vi "THzTime_SPEED_control_for Varying Gap_170120.vi"(1 "ESP300 Axis":i8=1, 2 "ESP300 Address":string="1", 4 "Lockin Address":string="12") -> ()   [LabVIEW 2010]
panel:
  in  "?":bool
  out "Current Round":i32=100
  out "Current Gap (um)":u32=50
  in  "Initial Gap (um)":u32=50
  out "error out":errorcluster
  in  "Number of Gap":u32=5
  in  "Number of Avg":u32=50
  in  "Gap Increase (um)":u32=25
  in  "Step Increase (um)":u32=5
  in  "error in (no error)":errorcluster
  in  "MCS System Locator":string="usb:id:1441320285"
  out "Y position":dbl=-0.3427166666666667 format="%#.3p"
  out "X position":dbl=-0.44846666666666674 format="%#.3p"
  out "Power meter":dbl=48.63333333333333 format="%#.3p"
  in  "Save File Name":string="vg_"
  in  "Launch server?":bool
  in  "Authorize?":bool=TRUE
  in  "CONEX-PSD9 Instrument Key 2":string="CONEX-PSD (A6ULD73M)"
  in  "Interdelay (ms)":dbl=20.0
  in  "pre delay(ms)":dbl=300.0
  out "Lock-in Y-Channel":dbl=7.27601e-12 format="%#.3p"
  out "Lock-in X-Channel":dbl=7.27601e-12 format="%#.3p"
  out "THz Time-domain Signal Wave":cluster{"x-axis":sgl[], "y-axis":dbl[]}(graph)
  in  "Autosave Directory for Long-term Average Scan":path=path "D:/taianh/Measurement Data/170121 Variable Gap"
  out "Phase":cluster{"f0":dbl, "df":dbl, "magnitude":dbl[]}(graph)
  in  "OK Button":bool
  out "Data Type":string="outp ? 1"
  in  "Enum":enum16{"X", "Y", "Abs"}(ring)
  in  "Draw":bool
  in  "Exit Program":bool
  out "Amplitude":cluster{"f0":dbl, "df":dbl, "magnitude":dbl[]}(graph)
  in  "Short term \nAverage#":i8=1
  in  "Step":sgl=0.005 min=0 max=10000 format="%.3f"
  in  "End Position":sgl=-18.5 min=-75 max=75 format="%#.3f"
  in  "Start Position":sgl=-16.2 min=-75 max=75 format="%#.3f"
  # "Data"
  # "Auto-offset"
  # "Start Position (mm)"
  # "End Position (mm)"
  # "Step (mm)"
  # "Point Avg"
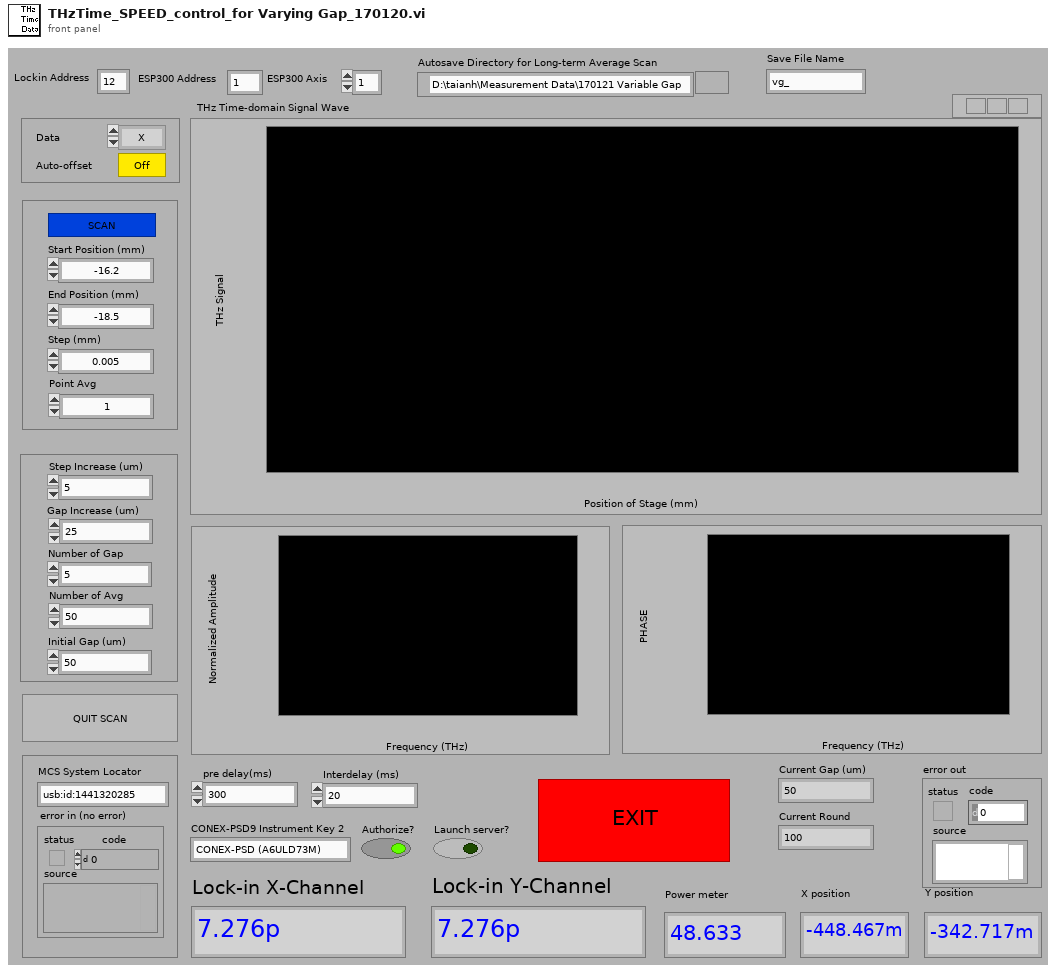
[diagram p1: front panel]
types:
  T1 = cluster{"ConexPSD Reference":refnum<k24>, "error out":errorcluster, "Component ID":i32}
  T2 = cluster{"System Index Out":u32, "error out":errorcluster}
  T3 = cluster{"Step Number":i32, "Step":sgl, "Start Position":sgl, "Time-out":i32, "Lockin Address":string, "Short term \nAverage#":i8, i32, "ESP300 Axis":i8, "Value":string, "pre delay(ms)":dbl, "Interdelay (ms)":dbl, "Autosave Directory for Long-term Average Scan":path, cluster{"ConexPSD Reference":refnum<k24>, "error out":errorcluster, "Component ID":i32}}
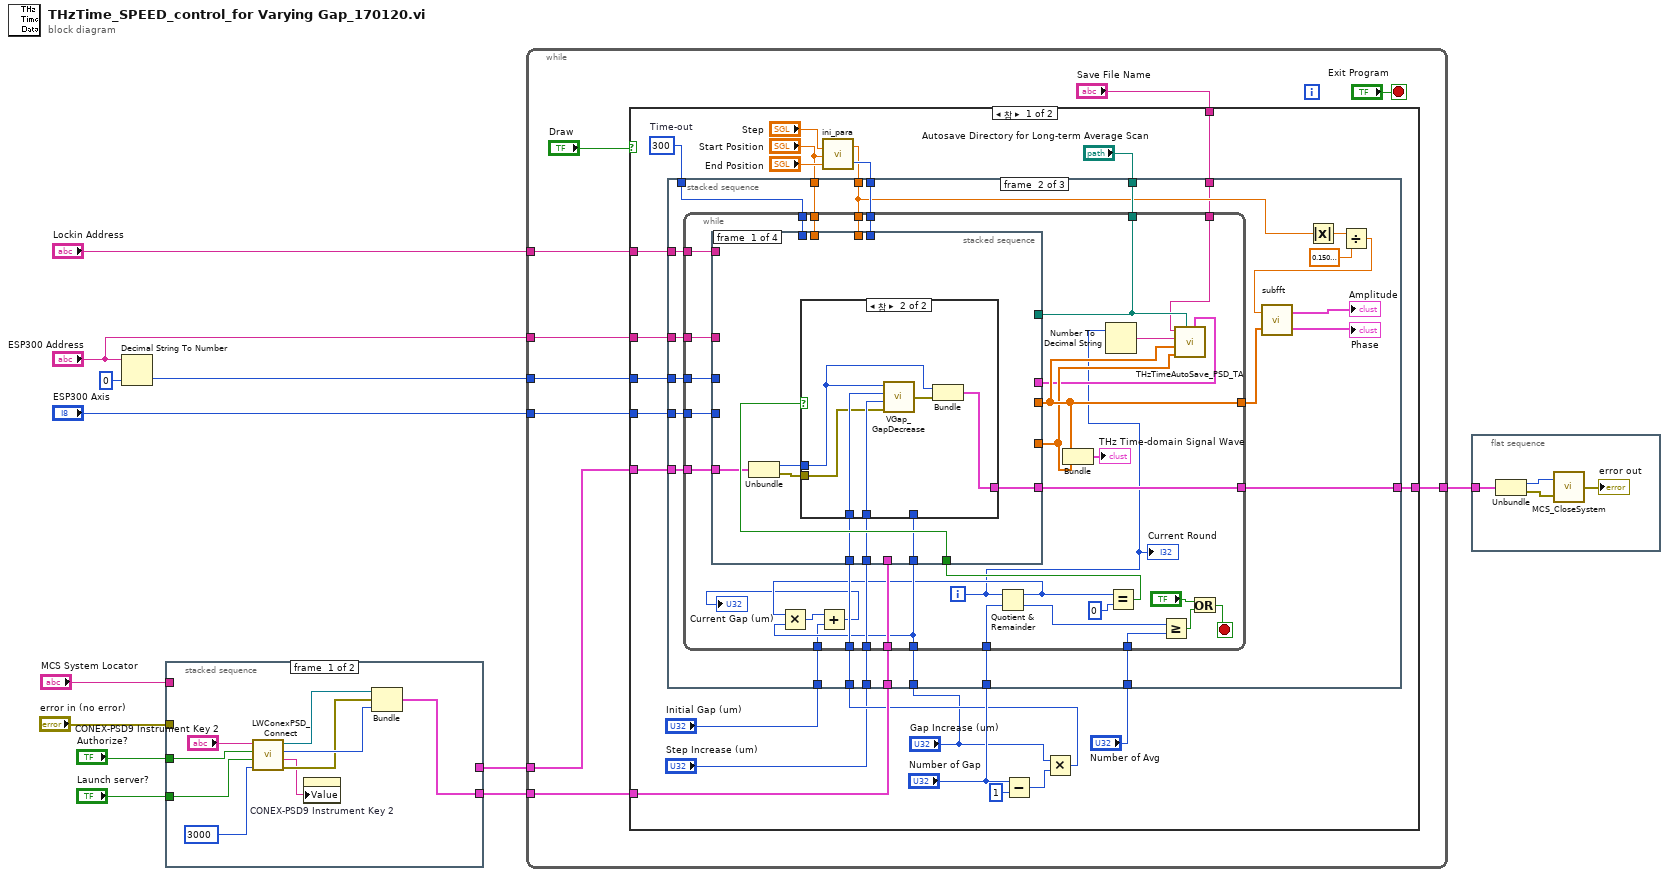
[diagram p0: block diagram]
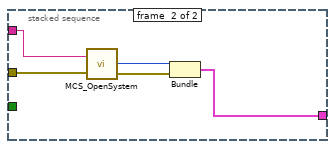
[diagram p2: hidden frame]
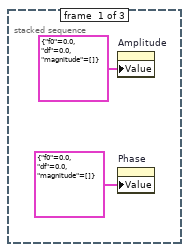
[diagram p3: hidden frame]
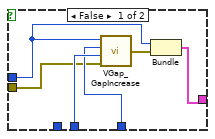
[diagram p4: hidden frame]
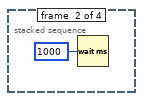
[diagram p5: hidden frame]
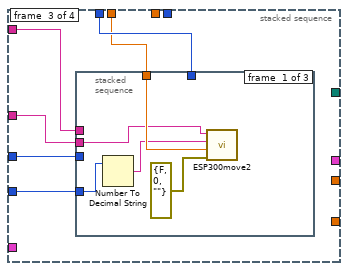
[diagram p6: hidden frame]
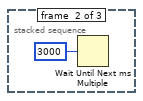
[diagram p7: hidden frame]
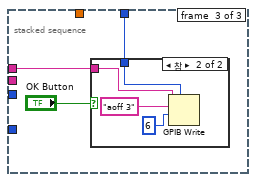
[diagram p8: hidden frame]
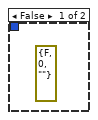
[diagram p9: hidden frame]
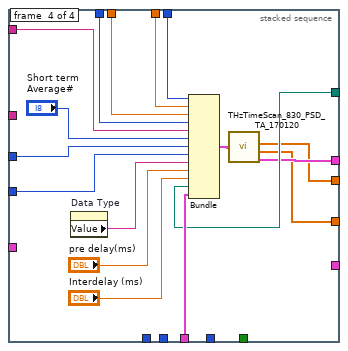
[diagram p10: hidden frame]
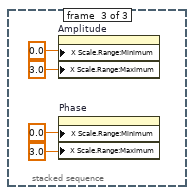
[diagram p11: hidden frame]
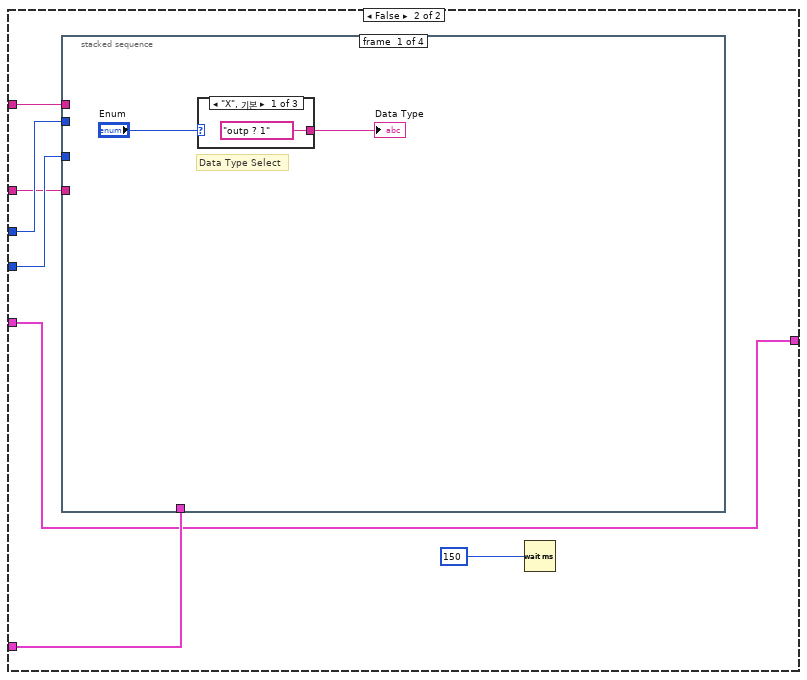
[diagram p12: hidden frame]
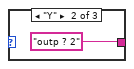
[diagram p13: hidden frame]
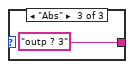
[diagram p14: hidden frame]
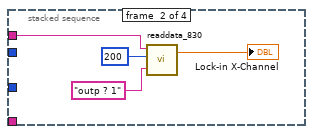
[diagram p15: hidden frame]
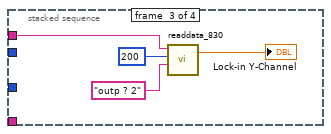
[diagram p16: hidden frame]
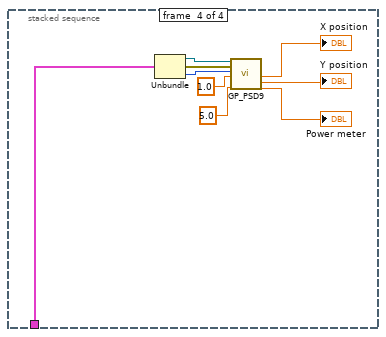
[diagram p17: hidden frame]
diagram:
  n1 = Decimal String To Number(string="ESP300 Address", default (0L)=0 ("default (0 I32)")) -> (number=w10:i32)  [unwired: 1 in, 1 out]
  n2 = stacked-sequence {
    tunnel: "Authorize?" -> [w15 _]
    tunnel: [w14 _] -> w5
    tunnel: "Launch server?" -> [w13 _]
    tunnel: "MCS System Locator" -> [_ w26]
    tunnel: "error in (no error)" -> [_ w25]
    tunnel: [_ w22] -> w2
    frame #0 {
      n3 = call "LWConexPSD_Connect.vi"("DiscoverTimeout (10000 msec)"=3000, "Launch server? (True)"=w13, "Authorize? (True)"=w15, "Instrument Key"="CONEX-PSD9 Instrument Key 2") -> ("error out"=w19:errorcluster, "Instrument Key out"=w17:string, "Component ID"=w20:i32, "ConexPSD Reference"=w18:refnum<k24>)
      n4 = property on="CONEX-PSD9 Instrument Key 2" class="Str"("Value"=w17) -> ()  [unwired: 2 in, 2 out]
      n5 = Bundle("ConexPSD Reference"=w18, "error out"=w19, "Component ID"=w20) -> (w14:T1)  [unwired: 1 in]
    }
    frame #1 {
      n6 = call "MCS_OpenSystem.vi"("error in (no error)"=w25, "MCS System Locator"=w26) -> ("error out"=w23:errorcluster, "System Index Out"=w24:u32)
      n7 = Bundle("System Index Out"=w24, "error out"=w23) -> (w22:T2)  [unwired: 1 in]
    }
  }
  n8 = while {
    tunnel: "ESP300 Axis" -> [w34]
    tunnel: "Lockin Address" -> [w33]
    tunnel: w10 -> [w32]
    tunnel: "ESP300 Address" -> [w31]
    tunnel: w5 -> [w30]
    tunnel: w2 -> [w28]
    tunnel: [w27] -> w1
    stop <- "Exit Program" stop-if-true
    n9 = case shown="참" "Draw" {
      tunnel: w33 -> [w59 w186]
      tunnel: w34 -> [w58 w188]
      tunnel: w32 -> [w57 w187]
      tunnel: w31 -> [w49 w184]
      tunnel: w30 -> [w48 w183]
      tunnel: "Save File Name" -> [w47 _]
      tunnel: w28 -> [w46 w182]
      tunnel: [w38 w182] -> w27
      frame True {
        w56 = 300  # Time-out
        n10 = call "ini_para.vi"("End Position"="End Position", "Start Position"="Start Position", "Step"="Step") -> ("Step Number"=w53:i32, "Step"=w52:sgl)
        n11 = Subtract(x="Number of Gap", y=u32 1) -> (x-y=w43:u32)
        n12 = Multiply(x="Gap Increase (um)", y=w43) -> (x*y=w42:u32)
        n13 = stacked-sequence {
          tunnel: w59 -> [_ w86 _]
          tunnel: w56 -> [_ w85 _]
          tunnel: w58 -> [_ w84 _]
          tunnel: w57 -> [_ w83 _]
          tunnel: w53 -> [_ w81 _]
          tunnel: w52 -> [_ w75 _]
          tunnel: "Start Position" -> [_ w82 _]
          tunnel: "Autosave Directory for Long-term Average Scan" -> [_ w80 _]
          tunnel: w49 -> [_ w73 _]
          tunnel: w48 -> [_ w72 _]
          tunnel: w47 -> [_ w71 _]
          tunnel: "Number of Gap" -> [_ w69 _]
          tunnel: w46 -> [_ w68 _]
          tunnel: w42 -> [_ w67 _]
          tunnel: "Step Increase (um)" -> [_ w66 _]
          tunnel: "Gap Increase (um)" -> [_ w65 _]
          tunnel: "Number of Avg" -> [_ w64 _]
          tunnel: [_ w63 _] -> w38
          tunnel: "Initial Gap (um)" -> [_ w62 _]
          frame #0 {
            n14 = property on="Amplitude" class="WFGraph (엄격한)"("Value"=cluster{"f0":dbl, "df":dbl, "magnitude":dbl[]} {"f0"=0.0, "df"=0.0, "magnitude"=[]} ("Spectrum")) -> ()  [unwired: 2 in, 2 out]
            n15 = property on="Phase" class="WFGraph (엄격한)"("Value"=cluster{"f0":dbl, "df":dbl, "magnitude":dbl[]} {"f0"=0.0, "df"=0.0, "magnitude"=[]} ("Spectrum")) -> ()  [unwired: 2 in, 2 out]
          }
          frame #1 {
            n16 = while {
              tunnel: w85 -> [w119]
              tunnel: w86 -> [w120]
              tunnel: w84 -> [w118]
              tunnel: w83 -> [w117]
              tunnel: w82 -> [w116]
              tunnel: w75 -> [w115]
              tunnel: w81 -> [w114]
              tunnel: w80 -> [w107]
              tunnel: [w109] -> w70
              tunnel: w73 -> [w112]
              tunnel: w72 -> [w111]
              tunnel: w71 -> [w106]
              tunnel: w69 -> [w104]
              tunnel: w68 -> [w101]
              tunnel: w67 -> [w97]
              tunnel: w66 -> [w100]
              tunnel: w65 -> [w96]
              tunnel: w64 -> [w99]
              tunnel: [w98] -> w63
              tunnel: w62 -> [w92]
              i -> [w94]
              stop <- w87 stop-if-true
              n17 = Quotient & Remainder(x=w94, y=w104) -> (x-y*floor(x/y)=w95:u32, floor(x/y)=w93:u32)
              n18 = Multiply(x=w95, y=w96) -> (x*y=w91:u32)
              n19 = Add(x=w91, y=w92) -> (x+y=→"Current Gap (um)":u32)
              n20 = Number To Decimal String(number=w94) -> (decimal integer string=w110:string)  [unwired: 1 in]
              n21 = Equal?(x=w95, y=u32 0) -> (x = y?=w102:bool)
              n22 = stacked-sequence {
                tunnel: w120 -> [_ _ w147 w173]
                tunnel: w119 -> [_ _ w146 w174]
                tunnel: w118 -> [_ _ w145 w170]
                tunnel: w117 -> [_ _ w144 w171]
                tunnel: w116 -> [_ _ w143 w175]
                tunnel: w115 -> [_ _ _ w176]
                tunnel: w114 -> [_ _ _ w177]
                tunnel: [_ _ _ w162] -> w109
                tunnel: [_ _ _ w161] -> w108
                tunnel: w112 -> [_ _ w142 _]
                tunnel: w107 -> [_ _ _ w165]
                tunnel: w111 -> [_ _ _ w166]
                tunnel: [_ _ _ w163] -> w105
                tunnel: w102 -> [w128 _ _ _]
                tunnel: w101 -> [w124 _ _ _]
                tunnel: w97 -> [w127 _ _ _]
                tunnel: w100 -> [w126 _ _ _]
                tunnel: w96 -> [w125 _ _ _]
                tunnel: [w121 _ _ _] -> w98
                frame #0 {
                  n23 = Unbundle(w124) -> ("System Index Out"=w122:u32, "error out"=w123:errorcluster)
                  n24 = case shown="참" w128 {
                    tunnel: w127 -> [_ w140]
                    tunnel: w126 -> [w134 w139]
                    tunnel: w125 -> [w133 _]
                    tunnel: w122 -> [w130 w136]
                    tunnel: w123 -> [w132 w138]
                    tunnel: [w129 w135] -> w121
                    frame False {
                      n25 = call "VGap_GapIncrease.vi"("error in (no error)"=w132, "Step Increase (um)"=w134, "Gap Increase (um)"=w133, "System Index In"=w130) -> ("error out"=w131:errorcluster)
                      n26 = Bundle("System Index Out"=w130, "error out"=w131) -> (w129:T2)  [unwired: 1 in]
                    }
                    frame True {
                      n27 = call "VGap_GapDecrease.vi"("error in (no error)"=w138, "Step Decrease (um)"=w139, "Gap Decrease (um)"=w140, "System Index In"=w136) -> ("error out"=w137:errorcluster)
                      n28 = Bundle("System Index Out"=w136, "error out"=w137) -> (w135:T2)  [unwired: 1 in]
                    }
                  }
                }
                frame #1 {
                  n29 = Wait (ms)(milliseconds to wait=u32 1000 ("대기 시간(ms)")) -> ()  [unwired: 1 out]
                }
                frame #2 {
                  n30 = stacked-sequence {
                    tunnel: w147 -> [_ _ w155]
                    tunnel: w146 -> [_ _ w154]
                    tunnel: w145 -> [w149 _ _]
                    tunnel: w144 -> [_ _ _]
                    tunnel: w143 -> [w152 _ _]
                    tunnel: w142 -> [w150 _ _]
                    frame #0 {
                      n31 = Number To Decimal String(number=w149) -> (decimal integer string=w148:string)  [unwired: 1 in]
                      n32 = call "ESP300move2.vi"("ESP300 Address"=w150, "ESP300 Channel"=w148, "Target"=w152, "error in (no error) 2"=errorcluster {"status"=FALSE, "code"=0, "source"=""}) -> ()  [unwired: 6 in, 1 out]
                    }
                    frame #1 {
                      n33 = Wait Until Next ms Multiple(millisecond multiple=3000) -> ()  [unwired: 1 out]
                    }
                    frame #2 {
                      n34 = case shown="참" "OK Button" {
                        tunnel: w155 -> [_ w160]
                        tunnel: w154 -> [_ w158]
                        frame False {
                          (unwired) errorcluster {"status"=FALSE, "code"=0, "source"=""} ("error in")
                        }
                        frame True {
                          n35 = GPIB Write(0:w160, 1:"aoff 3" ("data"), 2:i16 6 ("mode (0)"), 4:w158) -> ()  [unwired: 1 in, 2 out]
                        }
                      }
                    }
                  }
                }
                frame #3 {
                  n36 = property on="Data Type" class="Str"() -> ("Value"=w169:string)  [unwired: 2 in, 2 out]
                  n37 = Bundle("Step Number"=w177, "Step"=w176, "Start Position"=w175, "Time-out"=w174, "Lockin Address"=w173, "Short term \nAverage#"="Short term \nAverage#", w171, "ESP300 Axis"=w170, "Value"=w169, "pre delay(ms)"="pre delay(ms)", "Interdelay (ms)"="Interdelay (ms)", "Autosave Directory for Long-term Average Scan"=w165, w166) -> (w164:T3)  [unwired: 1 in]
                  n38 = call "THzTimeScan_830_PSD_TA_170120.vi"("input"=w164) -> ("x-axis"=w162:sgl[], "y-axis"=w161:dbl[], "ext. out"=w163:cluster{dbl[], dbl[], dbl[], dbl[], string[]})  [unwired: 1 out]
                }
              }
              n39 = Bundle("x-axis"=w109, "y-axis"=w108) -> (→"THz Time-domain Signal Wave":cluster{"x-axis":sgl[], "y-axis":dbl[]})  [unwired: 1 in]
              n40 = Greater Or Equal?(x=w93, y=w99) -> (x >= y?=w88:bool)
              n41 = call "THzTimeAutoSave_PSD_TA.vi"("ext. out"=w105, "Autosave Directory for Long-term Average Scan"=w107, "y-axis"=w108, "x-axis"=w109, "String"=w110, "SaveFile name"=w106) -> ()  [unwired: 4 in]
              n42 = Or(x="?", y=w88) -> (x .or. y?=w87:bool)
              "Current Round" <- w94
            }
            n43 = Absolute Value(x=w75) -> (abs(x)=w76:sgl)
            n44 = Divide(x=w76, y=sgl 0.15) -> (x/y=w74:sgl)
            n45 = call "subfft.vi"("y-signal"=w70, "time step"=w74) -> ("Phase"=→"Phase":cluster{"f0":dbl, "df":dbl, "real part":dbl[]}, "Amplitude"=→"Amplitude":cluster{"f0":dbl, "df":dbl, "real part":dbl[]})
          }
          frame #2 {
            n46 = property on="Amplitude" class="WFGraph (엄격한)"("X Scale.Range:Minimum"=0.0 ("X Scale.Range:Maximum"), "X Scale.Range:Maximum"=3.0) -> ()  [unwired: 2 in, 2 out]
            n47 = property on="Phase" class="WFGraph (엄격한)"("X Scale.Range:Minimum"=0.0, "X Scale.Range:Maximum"=3.0) -> ()  [unwired: 2 in, 2 out]
          }
        }
      }
      frame False {
        n48 = stacked-sequence {
          tunnel: w188 -> [_ _ _ _]
          tunnel: w187 -> [_ _ _ _]
          tunnel: w186 -> [_ w197 w201 _]
          tunnel: w184 -> [_ _ _ _]
          tunnel: w183 -> [_ _ _ w202]
          frame #0 {
            # "Data Type Select"
            n49 = case shown="\"X\", 기본" "Enum" {
              tunnel: ["outp ? 1" "outp ? 2" "outp ? 3"] -> w190
              frame "X", Default {
              }
              frame "Y" {
              }
              frame "Abs" {
              }
            }
            "Data Type" <- w190
          }
          frame #1 {
            n50 = call "readdata_830.vi"("Command"="outp ? 1", "timeout"=200, "Lockin Address"=w197) -> ("Data"=→"Lock-in X-Channel":dbl)  [unwired: 1 in, 1 out]
          }
          frame #2 {
            n51 = call "readdata_830.vi"("Command"="outp ? 2", "timeout"=200, "Lockin Address"=w201) -> ("Data"=→"Lock-in Y-Channel":dbl)  [unwired: 1 in, 1 out]
          }
          frame #3 {
            n52 = Unbundle(w202) -> ("ConexPSD Reference"=w210:refnum<k24>, "error out"=w209:errorcluster, "Component ID"=w208:i32)
            n53 = call "GP_PSD9.vi"("ConexPSD Reference"=w210, "error out"=w209, "Component ID"=w208, "Adress"=1.0 ("shot average"), "shot average"=5.0) -> ("PositionX"=→"X position":dbl, "PositionY"=→"Y position":dbl, "LaserPower"=→"Power meter":dbl)  [unwired: 8 in, 4 out]
          }
        }
        n54 = Wait (ms)(milliseconds to wait=u32 150) -> ()  [unwired: 1 out]
      }
    }
  }
  n55 = flat-sequence {
    tunnel: w1 -> [w214]
    frame #0 {
      n56 = Unbundle(w214) -> ("System Index Out"=w213:u32, "error out"=w212:errorcluster)
      n57 = call "MCS_CloseSystem.vi"("error in (no error)"=w212, "System Index In"=w213) -> ("error out"=→"error out":errorcluster)
    }
  }
